vi "GLOBALStateTest (1).vi"() -> ()   [LabVIEW 2017]
panel:
  in  "Magnetic Brake Pressure (PSI)":dbl
  in  "Suspension Pressure (PSI)":dbl
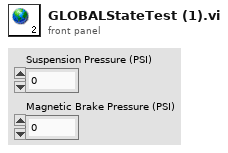
[diagram p1: front panel]
diagram:
